vi "parentWidget.vi"(8 "Error In":errorcluster, 11 "QLayout In":refnum<class "QLayout.lvclass">) -> (0 "Error Out":errorcluster, 2 "Value":refnum<class "QWidget.lvclass">, 3 "QLayout Out":refnum<class "QLayout.lvclass">)   [LabVIEW 2014, in "QLayout.lvclass"]
doc: "LabVIEW-specific documentation is not yet available. See <b>https://doc.qt.io/qt-5/qlayout.html#parentWidget</b>"
uses:
  QLayout.lvclass
  QWidget/QWidget.lvclass
  LQ Core/LQIdentity/LQIdentity.lvclass/LQIdentity.ctl
  LQ Core/LQ Core.lvlib
  LQ Core/LQIdentity/LQIdentity.lvclass
  LQ Core/LQCoreEngine/LQCoreEngine.lvclass
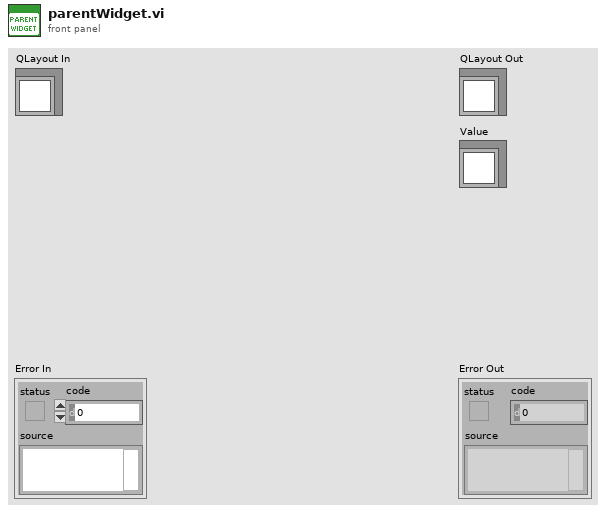
[diagram p1: front panel]
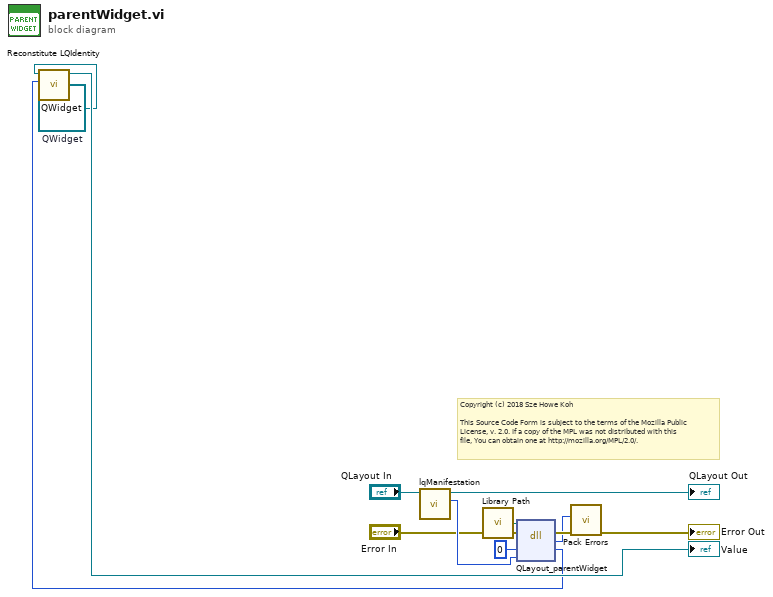
[diagram p0: block diagram]
diagram:
  w1 = refnum<class "QWidget.lvclass"> refnum  # QWidget
  # "Copyright (c) 2018 Sze Howe Koh\n\nThis Source Code Form is subject to the terms of the Mozilla Public\nLicense, v. 2.0. If a copy of the MPL was not distributed with this\nfile, You can obtain one at http://mozilla.org/MPL/2.0/."
  n1 = call "lqManifestation.vi"("LQIdentity in"="QLayout In") -> ("Manifestation"=w8:u64, "LQIdentity out"=→"QLayout Out":refnum<class "QLayout.lvclass">)  [unwired: 9 in]
  n2 = call "Library Path.vi"() -> ("Library Path"=w9:path)
  n3 = dll-call lib="?" fn="QLayout_parentWidget"(path in=w9, error in="Error In", "_retVal"=u64 0 ("retVal"), "_instance"=w8) -> (error out=w6:errorcluster, w4:i32, "_retVal"=w2:u64)  [unwired: 2 in, 1 out]
  n4 = call "Reconstitute LQIdentity.vi"("Manifestation"=w2, "LQIdentity Prototype"=w1) -> ("Reconstituted LQIdentity"=→"Value":refnum<class "QWidget.lvclass">)  [unwired: 8 in, 1 out]
  n5 = call "Pack Errors.vi"("Error In"=w6, "Error Code"=w4) -> ("Error Out"=→"Error Out":errorcluster)  [unwired: 9 in]
